vi "Execute Error Handling.vi"(8 "error in (no error)":errorcluster, 9 "Error":errorcluster, 10 "Error Level":T1, 11 "Elevator Controller Actor in":refnum<class "Elevator Controller Actor.lvclass">) -> (0 "error out":errorcluster, 3 "Elevator Controller Actor out":refnum<class "Elevator Controller Actor.lvclass">)   [LabVIEW 2022 SP3, in "Elevator Controller Actor.lvlib" / "Elevator Controller Actor.lvclass"]
uses:
  Elevator Controller Actor.lvclass
  Elevator Controller Actor.lvclass/Elevator Controller Actor.ctl
  Interface Elevator/Interface Elevator Msg/Set State Msg/Set State Msg.lvclass
  <vilib>/ActorFramework/Actor/Actor.lvclass
  State -Enum.ctl
  Error Level.ctl
  Log Data.ctl
  C:/Program Files/National Instruments/LabVIEW 2022/vi.lib/ActorFramework/Actor/Actor.lvclass
  C:/Workspace/CLA/Elevator AF_2022_2nd/Elevator Controller Actor/Elevator Controller Actor/Elevator Controller Actor.lvclass
  C:/Workspace/CLA/Elevator AF_2022_2nd/Interface Elevator/Interface Elevator/Interface Elevator.lvclass
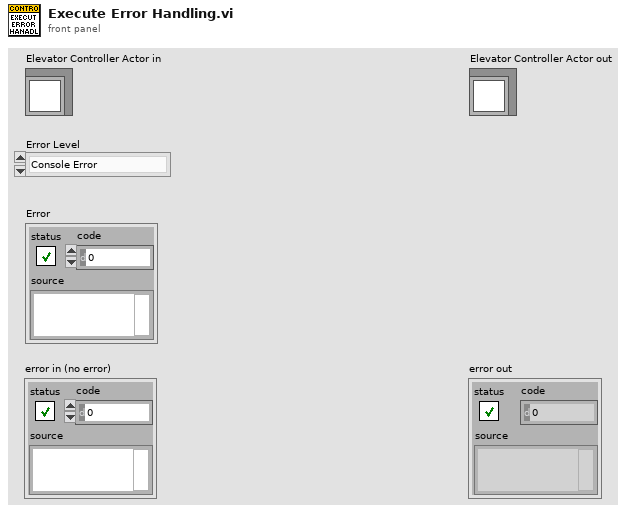
[diagram p1: front panel]
types:
  T1 = typedef "Elevator Controller Actor.lvlib/Elevator Controller Actor.lvclass/Error Level.ctl" = enum16{"Console Error", "Sensor Interface IO Error", "Process Step Error"}
  T2 = typedef "Elevator Controller Actor.lvlib/Elevator Controller Actor.lvclass/Log Data.ctl" = cluster{"Description":string, "Error Level":T1, "Time Stamp":timestamp}
  T3 = typedef "Elevator Controller Actor.lvlib/Elevator Controller Actor.lvclass/State -Enum.ctl" = enum16{"Initial", "Wait for First Request", "Start and Move", "Anaysis", "Continue Travel", "Stop at Floor", "Open and Close Door Sequence", "No Request Remaining", "Emergency Call", "Terminate Process"}
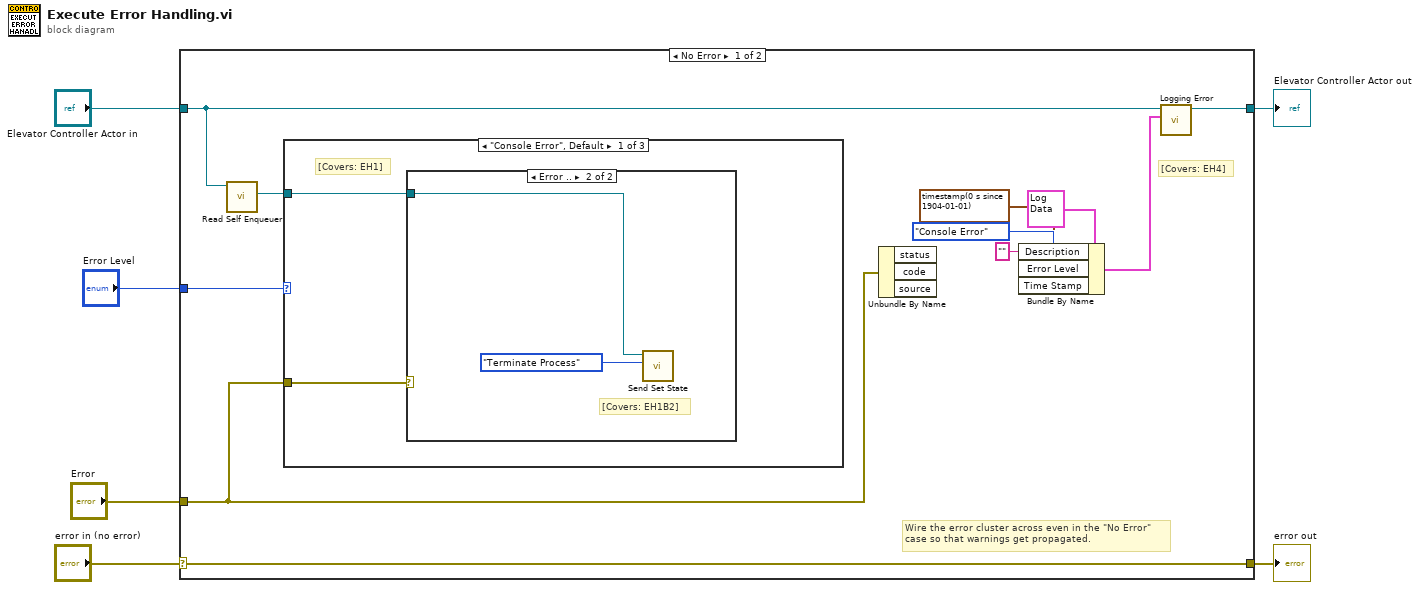
[diagram p0: block diagram]
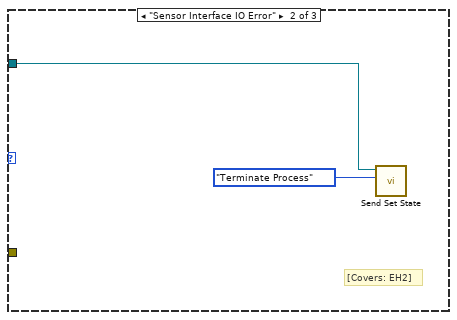
[diagram p3: hidden frame]
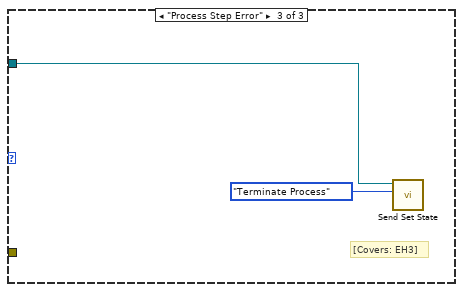
[diagram p4: hidden frame]
diagram:
  n1 = case shown="No Error" "error in (no error)" {
    selector: "error in (no error)" -> [w17 w27]
    tunnel: [w17 w27] -> w5
    tunnel: [w13 w26] -> w3
    tunnel: "Elevator Controller Actor in" -> [w14 w26]
    tunnel: "Error Level" -> [w16 _]
    tunnel: "Error" -> [w10 _]
    frame No Error {
      # "[Covers: EH4]"
      # "Wire the error cluster across even in the \"No Error\"\ncase so that warnings get propagated."
      n2 = call <vilib>:"Read Self Enqueuer.vi"("Actor"=w14) -> ("Self Enqueuer"=w15:refnum<class "Message Enqueuer.lvclass">)  [unwired: 10 in]
      n3 = case shown="\"Console Error\", Default" w16 {
        tunnel: w15 -> [w18 w23 w24]
        tunnel: w10 -> [w19 _ _]
        frame "Console Error", Default {
          # "[Covers: EH1]"
          n4 = case shown="Error .." w19 {
            tunnel: w18 -> [_ w20]
            frame No Error {
              # "[Covers: EH1B1]"
            }
            frame Error {
              # "[Covers: EH1B2]"
              n5 = call "Send Set State.vi"("State"=State_-Enum."Terminate Process", "Message Enqueuer"=w20) -> ()  [unwired: 8 in, 2 out]
            }
          }
        }
        frame "Sensor Interface IO Error" {
          # "[Covers: EH2]"
          n6 = call "Send Set State.vi"("State"=State_-Enum."Terminate Process", "Message Enqueuer"=w23) -> ()  [unwired: 8 in, 2 out]
        }
        frame "Process Step Error" {
          # "[Covers: EH3]"
          n7 = call "Send Set State.vi"("State"=State_-Enum."Terminate Process", "Message Enqueuer"=w24) -> ()  [unwired: 8 in, 2 out]
        }
      }
      n8 = Unbundle By Name(w10) -> ()  [unwired: 3 out]
      n9 = Bundle By Name(cluster=T2 {"Description"="", "Error Level"=enum."Console Error", "Time Stamp"=timestamp(0 s since 1904-01-01)} ("Log Data"), "Description"="", "Error Level"=Error_Level."Console Error", "Time Stamp"=timestamp(0 s since 1904-01-01)) -> (w12:T2)
      n10 = call "Logging Error.vi"("Log Data"=w12, "Elevator Controller Actor in"=w14) -> ("Elevator Controller Actor out"=w13:refnum<class "Elevator Controller Actor.lvclass">)  [unwired: 8 in, 1 out]
    }
    frame Error {
    }
  }
  "error out" <- w5
  "Elevator Controller Actor out" <- w3
